vi "Drop Marker.vi"(8 "error in (no error)":errorcluster, 11 "Mouse in":refnum<class "Mouse.lvclass">) -> (0 "error out":errorcluster, 3 "Mouse out":refnum<class "Mouse.lvclass">)   [LabVIEW 2020, in "Maze.lvlib" / "Mouse.lvclass"]
doc: "Drops a marker at the mouse's current location on the map. A location can only be marked once. If there is already a mark at this location then nothing happens. Markers can be checked for with <b>Check for Marker.vi</b> and removed with <b>Pickup Marker.vi</b> Using markers will score lower as it means an internal map is not being built within the mouse implementation."
uses:
  Mouse.lvclass
  Mouse.lvclass/Mouse.ctl
  Maze/Maze.lvclass
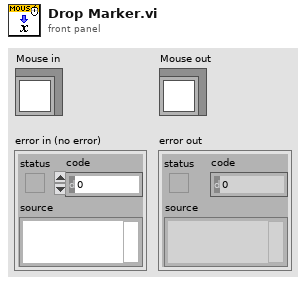
[diagram p1: front panel]
types:
  T1 = typedef "Maze.lvlib/Position.ctl" = cluster{"S":i32, "E":i32}
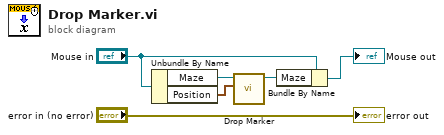
[diagram p0: block diagram]
diagram:
  n1 = Unbundle By Name("Mouse in") -> ("Maze"=w4:refnum<class "Maze.lvclass">, "Position"=w3:T1)
  n2 = call "Drop Marker.vi"("Position"=w3, "Maze in"=w4) -> ("Maze out"=w1:refnum<class "Maze.lvclass">)  [unwired: 8 in, 1 out]
  n3 = Bundle By Name(cluster="Mouse in", "Maze"=w1) -> (→"Mouse out":refnum<class "Mouse.lvclass">)
  "error out" <- "error in (no error)"
